vi "Parse Header.vi"(11 "body":string) -> (0 "Remaining String":string, 3 "Header Data":string[](array[string]))   [LabVIEW 2020]
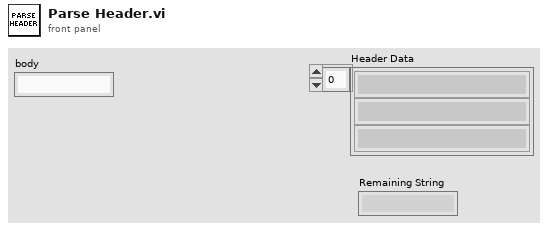
[diagram p1: front panel]
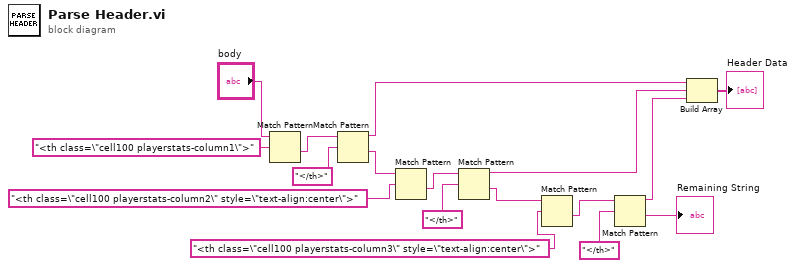
[diagram p0: block diagram]
diagram:
  n1 = Match Pattern(string="body", regular expression="<th class=\"cell100 playerstats-column1\">") -> (after substring=w8:string)  [unwired: 1 in, 3 out]
  n2 = Match Pattern(string=w8, regular expression="</th>") -> (before substring=w4:string, after substring=w10:string)  [unwired: 1 in, 2 out]
  n3 = Match Pattern(string=w10, regular expression="<th class=\"cell100 playerstats-column2\" style=\"text-align:center\">") -> (after substring=w12:string)  [unwired: 1 in, 3 out]
  n4 = Match Pattern(string=w12, regular expression="</th>") -> (before substring=w3:string, after substring=w15:string)  [unwired: 1 in, 2 out]
  n5 = Match Pattern(string=w15, regular expression="<th class=\"cell100 playerstats-column3\" style=\"text-align:center\">") -> (after substring=w16:string)  [unwired: 1 in, 3 out]
  n6 = Match Pattern(string=w16, regular expression="</th>") -> (before substring=w2:string, after substring=→"Remaining String":string)  [unwired: 1 in, 2 out]
  n7 = Build Array(w4, w3, w2) -> (→"Header Data":string[])
